vi "VariableGroupToCluster.vi"(11 "VariableGroup":refnum<class "VariableGroup.lvclass">) -> (3 "VariableGroupCluster":T1)   [LabVIEW 2012, in "VariableManagerAPI.lvlib"]
uses:
  VariableManagerAPI.lvlib
  VariableGroup/VariableGroup.lvclass
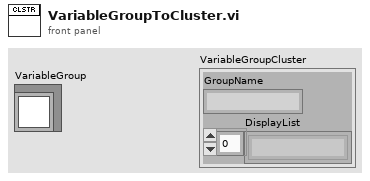
[diagram p1: front panel]
types:
  T1 = cluster{"GroupName":string, "DisplayList":string[]}
  T2 = cluster{"Accessors:GroupName":string, "Accessors:DisplayList":string[]}
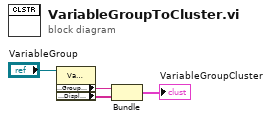
[diagram p0: block diagram]
diagram:
  n1 = property class="VariableGroup.lvclass"(reference="VariableGroup") -> ("Accessors:GroupName"=w3:string, "Accessors:DisplayList"=w2:string[])  [unwired: 1 in, 2 out]
  n2 = Bundle("Accessors:GroupName"=w3, "Accessors:DisplayList"=w2) -> (→"VariableGroupCluster":T2)  [unwired: 1 in]
